vi "SP VNA Cannot Measure SPs Warning.vi"(8 "error in (no error)":errorcluster, 11 "Removed Parameters":T1[](array[typedef]) {"Channel" min=1 max=99 step=1; "Parameter"."Stimulus Port" min=1 step=1; "Parameter"."Response Port" min=1 step=1}) -> (0 "error out":errorcluster, 3 "Choice":i32=2)   [LabVIEW 2011]
uses:
  TypeDefs/SP Parameter to Measure.ctl
  TypeDefs/SP Parameter.ctl
  TypeDefs/SP Calibration State.ctl
  TypeDefs/SP Measurement Format.ctl
panel:
  out "Message (\"\")":string="The following S Parameters cannot be measured by the instrument connected to this test station.\n\nDo you want to continue without measuring these S Parameters?"
  in  "Abort":bool
  in  "Continue":bool
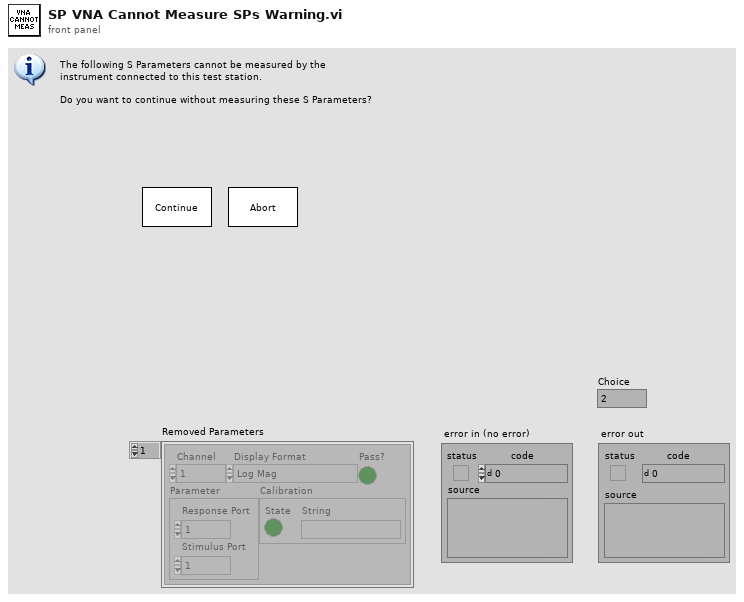
[diagram p1: front panel]
types:
  T1 = typedef "SP Parameter to Measure.ctl" = cluster{"Channel":i8, "Parameter":T2, "Calibration":T3, "Display Format":T4, "Pass?":bool}
  T2 = typedef "SP Parameter.ctl" = cluster{"Stimulus Port":i8, "Response Port":i8}
  T3 = typedef "SP Calibration State.ctl" = cluster{"State":bool, "String":string}
  T4 = typedef "SP Measurement Format.ctl" = enum32{"Log Mag", "Phase", "Delay", "Smith (R+jX)", "Polar (Re/Im)", "Linear Mag", "SWR", "Real", "Imaginary", "Smith (Lin/Phase)", "Smith (Log/Phase)", "Smith (Real/Imag)", "Smith (G+jB)", "Polar (Lin/Phase)", "Polar (Log/Phase)", "Expanded Phase", "Positive Phase", "Inverted Smith", "Unwrapped Phase", "Power Out", "Power In", "Linear Mag/Phase", "Log Mag/Phase", "Real/Imaginary"}
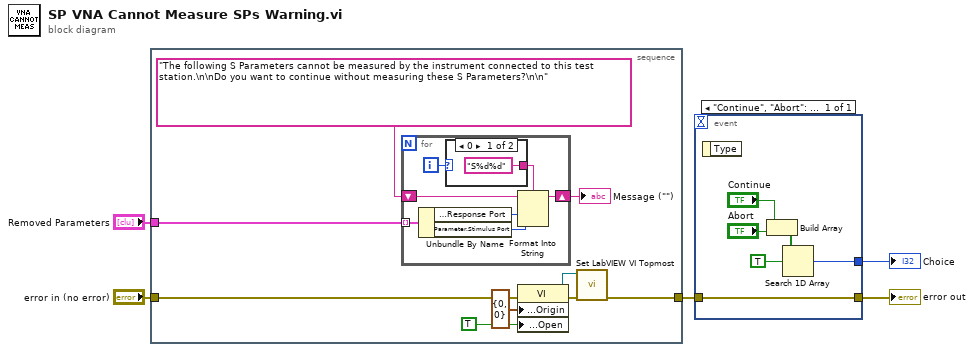
[diagram p0: block diagram]
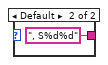
[diagram p2: hidden frame]
diagram:
  n1 = stacked-sequence {
    tunnel: "error in (no error)" -> [w14]
    tunnel: [w11] -> w1
    tunnel: "Removed Parameters" -> [w8]
    frame #0 {
      n2 = for {
        tunnel: w8 -> [w21] mode=indexing
        shift-right: [w18] -> w6
        shift-left: "The following S Parameters cannot be measured by the instrument connected to this test station.\n\nDo you want to continue without measuring these S Parameters?\n\n" ("Message (\"\")") -> [w17]
        i -> [w15]
        n3 = Unbundle By Name(w21) -> ("Parameter.Response Port"=w20:i8, "Parameter.Stimulus Port"=w19:i8)
        n4 = case shown="0" w15 {
          tunnel: ["S%d%d" ("format string") ", S%d%d" ("format string")] -> w16
          frame 0 {
          }
          frame Default {
          }
        }
        n5 = Format Into String(format string=w16, initial string=w17, w20, w19) -> (resulting string=w18:string)  [unwired: 1 in, 1 out]
      }
      "Message (\"\")" <- w6
      n6 = property on="Property Node" class="VI"(error in=w14, "Front Panel Window:Origin"=cluster{"Horizontal":i16, "Vertical":i16} {"Horizontal"=0, "Vertical"=0}, "Front Panel Window:Open"=TRUE) -> (reference out=w10:refnum<vi>, error out=w12:errorcluster)  [unwired: 1 in]
      n7 = call "Set LabVIEW VI Topmost.vi"("error in (no error)"=w12, "VI Refnum (null)"=w10) -> ("error out"=w11:errorcluster)  [unwired: 7 in, 2 out]
    }
  }
  n8 = event shown="[0] \"Continue\", \"Abort\": Value Change" {
    selector: _ -> [_]
    dyn-events: _ -> [_]
    timeout: _ -> [_]
    tunnel: w1 -> [w29]
    tunnel: [w29] -> w5
    tunnel: [w24] -> w4
    event "Continue", "Abort": Value Change {
      n9 = event-data() -> ()  [unwired: 2 out]
      n10 = Build Array("Continue", "Abort") -> (w26:bool[])
      n11 = Search 1D Array(1D array=w26, element=TRUE) -> (index of element=w24:i32)  [unwired: 1 out]
    }
  }
  "error out" <- w5
  "Choice" <- w4
